vi "Bool to Double.vi"(3 "Bool":bool) -> (1 "Double":dbl)   [LabVIEW 2020, in "Vecto.lvlib"]
uses:
  Vecto.lvlib
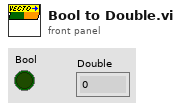
[diagram p1: front panel]
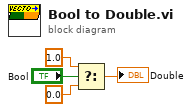
[diagram p0: block diagram]
diagram:
  n1 = Select(t=1.0, s="Bool", f=0.0) -> (s? t:f=→"Double":dbl)
